vi "ActDriveStraight.vi"(9 "FirstTime":bool, 10 "MaxSpeed (ft/s)":dbl, 11 "Dist (ft)":dbl) -> (0 "LeftSpeedDemand":dbl, 1 "Unfiltered Done Right":bool, 2 "Unfiltetred Done Left":bool, 3 "Done":bool, 4 "RightSpeedDemand":dbl)   [LabVIEW 2020]
doc: "Drive the robot straight in arcade drive\nList of things to tune:\n-MaxSpeed\n-ErrorThresh\n-ErrorDead\n-MinOutput\n-MaxOutput\n-Count\n\nInputs:\n--Dist -- Double -- in feet, the distance you want to go when you push the joystick (Get this value from human input)\n-- MaxSpeed -- Double -- in ft/s, the MaxSpeed the robot can go (NEEDS TO BE TUNED)\n-- First Time - Bool -- is this the first time the distance is changing? \n\nOutputs:\n-- Done -- Bool -- has the robot reached its target distance\n-- Unfilt. L Target -- Bool -- unfilteredOnTarget for Left, for debugging purposes\n-- Unfilt. R Target -- Bool -- unfilteredOnTarget for Right, for debugging purposes"
uses:
  <vilib>/Rock Robotics/Network Tables/NT Write Number.vi
  <vilib>/Rock Robotics/Network Tables/NT Write Boolean.vi
  <vilib>/Rock Robotics/WPI/ThirdParty/JAS_Junk/TrajLib/Trajectory_Library.lvlib
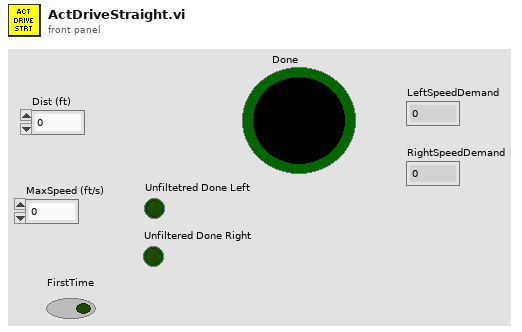
[diagram p1: front panel]
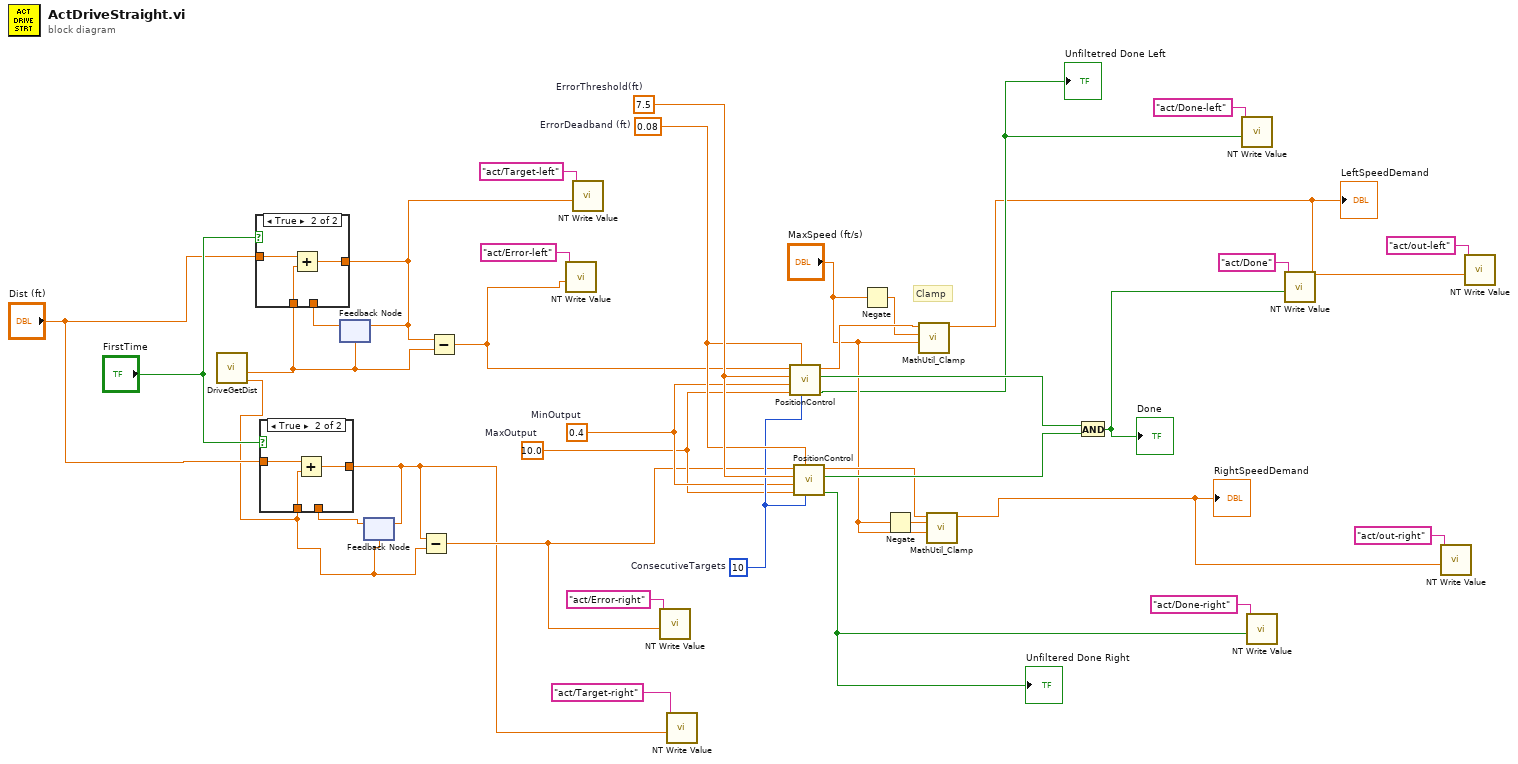
[diagram p0: block diagram]
diagram:
  w14 = 10.0  # MaxOutput
  w15 = 0.4  # MinOutput
  w28 = 10  # ConsecutiveTargets
  w31 = 0.08  # ErrorDeadband (ft)
  w32 = 7.5  # ErrorThreshold(ft)
  # "Clamp"
  n1 = call "DriveGetDist.vi"() -> ("Right dist"=w22:dbl, "Left dist"=w18:dbl)  [unwired: 10 in]
  n2 = feedback #1(w18) -> (w34:dbl)
  n3 = case shown="True" "FirstTime" {
    tunnel: "Dist (ft)" -> [_ w40]
    tunnel: w18 -> [_ w39]
    tunnel: [w37 w38] -> w20
    tunnel: w34 -> [w37 _]
    frame False {
    }
    frame True {
      n4 = Add(x=w40, y=w39) -> (x+y=w38:dbl)
    }
  }
  n5 = feedback-in #1(w20) -> ()
  n6 = feedback #2(w22) -> (w33:dbl)
  n7 = case shown="True" "FirstTime" {
    tunnel: "Dist (ft)" -> [_ w44]
    tunnel: w22 -> [_ w43]
    tunnel: [w41 w42] -> w9
    tunnel: w33 -> [w41 _]
    frame False {
    }
    frame True {
      n8 = Add(x=w44, y=w43) -> (x+y=w42:dbl)
    }
  }
  n9 = feedback-in #2(w9) -> ()
  n10 = Subtract(x=w9, y=w22) -> (x-y=w12:dbl)
  n11 = Subtract(x=w20, y=w18) -> (x-y=w11:dbl)
  n12 = call-poly <vilib>:"NT Write Value.vi"("value"=w11, "name"="act/Error-left") -> ()  [unwired: 9 in, 1 out]
  n13 = call-poly <vilib>:"NT Write Value.vi"("value"=w20, "name"="act/Target-left") -> ()  [unwired: 9 in, 1 out]
  n14 = call-poly <vilib>:"NT Write Value.vi"("value"=w12, "name"="act/Error-right") -> ()  [unwired: 9 in, 1 out]
  n15 = call-poly <vilib>:"NT Write Value.vi"("value"=w9, "name"="act/Target-right") -> ()  [unwired: 9 in, 1 out]
  n16 = call "PositionControl.vi"("ConsecutiveTargets"=w28, "ErrorDeadband"=w31, "MaxOutput"=w14, "MinOutput"=w15, "ErrorThreshold"=w32, "Error"=w11) -> ("UnfilteredOnTarget"=w5:bool, "OnTarget"=w29:bool, "OutputValue"=w27:dbl)  [unwired: 3 in]
  "Unfiltetred Done Left" <- w5
  n17 = call "PositionControl.vi"("ConsecutiveTargets"=w28, "ErrorDeadband"=w31, "MaxOutput"=w14, "MinOutput"=w15, "ErrorThreshold"=w32, "Error"=w12) -> ("UnfilteredOnTarget"=w6:bool, "OnTarget"=w30:bool, "OutputValue"=w25:dbl)  [unwired: 3 in]
  "Unfiltered Done Right" <- w6
  n18 = Negate(x="MaxSpeed (ft/s)") -> (-x=w26:dbl)
  n19 = Negate(x="MaxSpeed (ft/s)") -> (-x=w24:dbl)
  n20 = call <vilib>:"MathUtil_Clamp.vi"("High Limit"="MaxSpeed (ft/s)", "Low Limit"=w26, "Value"=w27) -> ("Result"=w3:dbl)  [unwired: 8 in]
  "LeftSpeedDemand" <- w3
  n21 = call <vilib>:"MathUtil_Clamp.vi"("High Limit"="MaxSpeed (ft/s)", "Low Limit"=w24, "Value"=w25) -> ("Result"=w1:dbl)  [unwired: 8 in]
  "RightSpeedDemand" <- w1
  n22 = And(x=w29, y=w30) -> (x .and. y?=w16:bool)
  "Done" <- w16
  n23 = call-poly <vilib>:"NT Write Value.vi"("value"=w5, "name"="act/Done-left") -> ()  [unwired: 9 in, 1 out]
  n24 = call-poly <vilib>:"NT Write Value.vi"("value"=w6, "name"="act/Done-right") -> ()  [unwired: 9 in, 1 out]
  n25 = call-poly <vilib>:"NT Write Value.vi"("value"=w16, "name"="act/Done") -> ()  [unwired: 9 in, 1 out]
  n26 = call-poly <vilib>:"NT Write Value.vi"("value"=w1, "name"="act/out-right") -> ()  [unwired: 9 in, 1 out]
  n27 = call-poly <vilib>:"NT Write Value.vi"("value"=w3, "name"="act/out-left") -> ()  [unwired: 9 in, 1 out]
